vi "XML Write.vi"() -> ()   [LabVIEW 2023]
uses:
  TAGS.ctl
panel:
  out "output cluster":cluster{"TAGLIST":T1[]}
  out "Array":cluster{"TAG":T1}[][](array[cluster])
  in  "TAG":T1[](array[typedef])
  out "output array 2":string[](array[string])
  in  "Schedule Filename":string
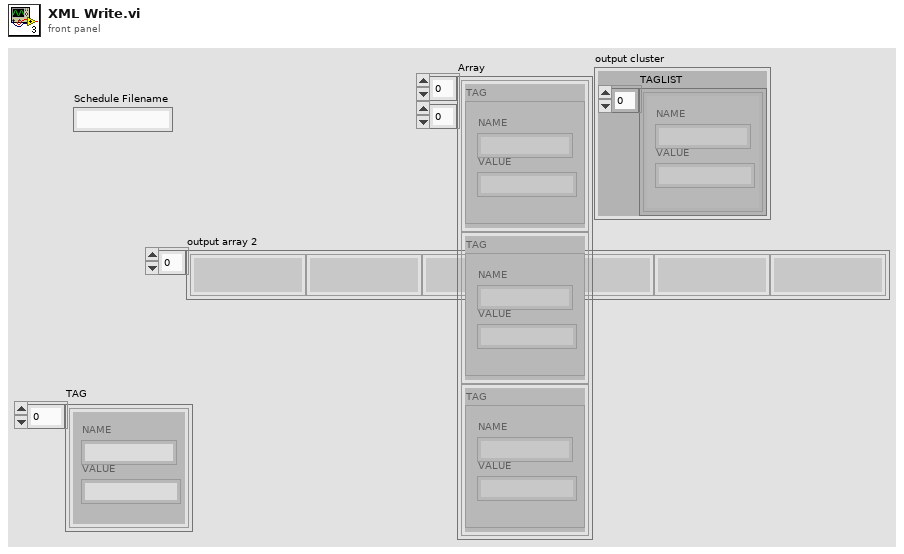
[diagram p1: front panel]
types:
  T1 = typedef "TAGS.ctl" = cluster{"NAME":string, "VALUE":string}
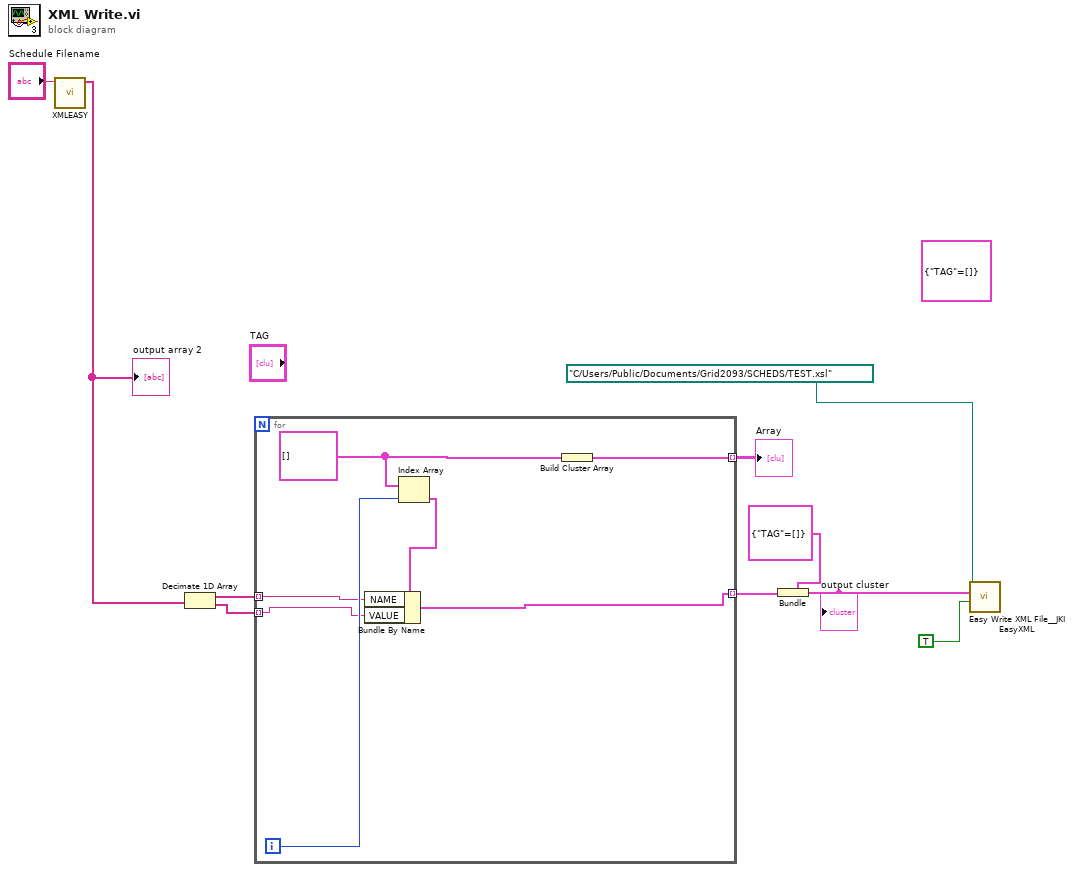
[diagram p0: block diagram]
diagram:
  (unwired) cluster{"TAG":cluster{"TAG":T1}[]} {"TAG"=[]} ("TAGLIST")
  n1 = call "XMLEASY.vi"("Schedule Filename"="Schedule Filename") -> ("output array"=w5:string[])  [unwired: 10 in]
  "output array 2" <- w5
  n2 = Decimate 1D Array(w5) -> (w8:string[], w9:string[])
  n3 = for {
    tunnel: w9 -> [w12] mode=indexing
    tunnel: w8 -> [w13] mode=indexing
    tunnel: [w11] -> w2 mode=indexing
    tunnel: [w17] -> w4 mode=indexing
    i -> [w15]
    w16 = T1[] [] ("TAG")
    n4 = Index Array(array=w16, index=w15) -> (element=w14:T1)
    n5 = Bundle By Name(cluster=w14, "NAME"=w13, "VALUE"=w12) -> (w11:T1)
    n6 = Build Cluster Array(w16) -> (w17:cluster{"TAG":T1}[])
  }
  "Array" <- w4
  n7 = Bundle(cluster=cluster{"TAG":T1[]} {"TAG"=[]} ("TAGLIST"), "TAG"=w2) -> (w3:cluster{"TAG":T1[]})
  "output cluster" <- w3
  n8 = call <vilib>:"Easy Write XML File__JKI EasyXML.vi"("Overwrite File? (false)"=TRUE, "LabVIEW Data"=w3, "XML File Path"=path "C:/Users/Public/Documents/Grid2093/SCHEDS/TEST.xsl") -> ()  [unwired: 7 in, 2 out]
